vi "Create.vi"(8 "error in (no error)":errorcluster, 10 "Instrument_type":T1="Toolbox") -> (0 "error out":errorcluster, 3 "_Driver_interaction out":refnum<class "_Driver_interaction.lvclass">)   [LabVIEW 2014, in "Driver_interaction.lvlib" / "_Driver_interaction.lvclass"]
uses:
  _Driver_interaction.lvclass
  Controls/Driver_interaction_instrument_type.ctl
  Toolbox/Toolbox.lvclass
  Dali_usb/Dali_usb_tridonics.lvclass
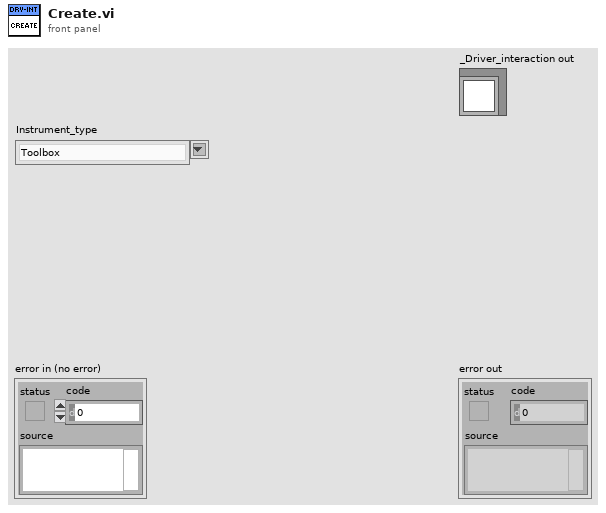
[diagram p1: front panel]
types:
  T1 = typedef "Driver_interaction.lvlib/_Driver_interaction.lvclass/Driver_interaction_instrument_type.ctl" = string
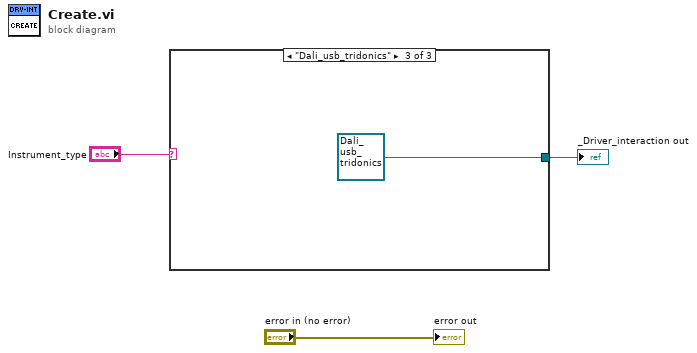
[diagram p0: block diagram]
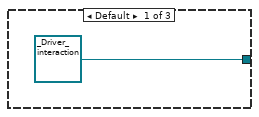
[diagram p2: hidden frame]
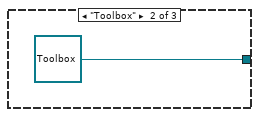
[diagram p3: hidden frame]
diagram:
  n1 = case shown="\"Dali_usb_tridonics\"" "Instrument_type" {
    tunnel: [refnum<class "_Driver_interaction.lvclass"> refnum ("_Driver_interaction out") refnum<class "Toolbox.lvclass"> refnum ("Driver_interaction.lvlib:Toolbox.lvclass") refnum<class "Dali_usb_tridonics.lvclass"> refnum ("Driver_interaction.lvlib:Dali_usb_tridonics.lvclass")] -> w1
    frame Default {
    }
    frame "Toolbox" {
    }
    frame "Dali_usb_tridonics" {
    }
  }
  "_Driver_interaction out" <- w1
  "error out" <- "error in (no error)"
